vi "Write slope type.vi"(8 "error in (no error)":errorcluster caption="에러 입력(에러 없음)", 10 "slope type":T1, 11 "Square Wave 입력":refnum<class "Square Wave.lvclass">) -> (0 "error out":errorcluster caption="에러 출력", 3 "Square Wave 출력":refnum<class "Square Wave.lvclass">)   [LabVIEW 2020, in "Square Wave.lvclass"]
uses:
  Square Wave.lvclass
  Controls/Slope Type.ctl
  Square Wave.lvclass/Square Wave.ctl
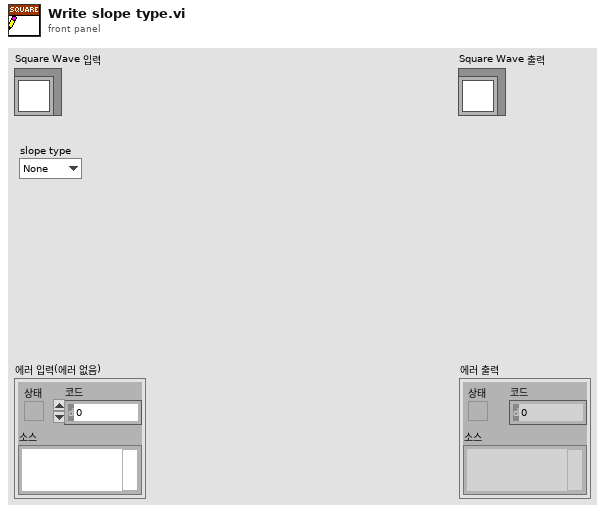
[diagram p1: front panel]
types:
  T1 = typedef "Square Wave.lvclass/Slope Type.ctl" = enum16{"None", "Lin.", "Exp."}
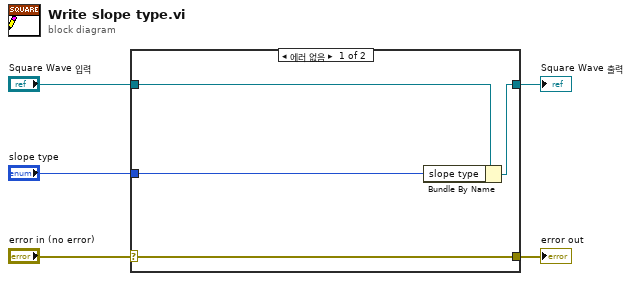
[diagram p0: block diagram]
diagram:
  n1 = case shown="에러 없음" "error in (no error)" {
    selector: "error in (no error)" -> [w9 w10]
    tunnel: [w9 w10] -> w4
    tunnel: [w7 w11] -> w2
    tunnel: "Square Wave 입력" -> [w8 w11]
    tunnel: "slope type" -> [w6 _]
    frame No Error {
      n2 = Bundle By Name(cluster=w8, "slope type"=w6) -> (w7:refnum<class "Square Wave.lvclass">)
    }
    frame Error {
    }
  }
  "error out" <- w4
  "Square Wave 출력" <- w2
